vi "myRIO_BRig_RT__Case_Exp_State_Reward__v2.vi"(0 "input_dataCurrent":u16[](array[numeric]), 5 "input_state":T1, 9 "input_spout":enum16{"Left", "Right"}(ring), 12 "input_dataExp":u16[](array[numeric]), 13 "input_dataTrial":u16[][](array[numeric])) -> (4 "output_dataCurrent":u16[](array[numeric]), 6 "output_state":T1, 8 "output__L":bool, 10 "output__R":bool)   [LabVIEW 2014]
uses:
  myRIO_BRig_RT__Case_Exp_stateList.ctl
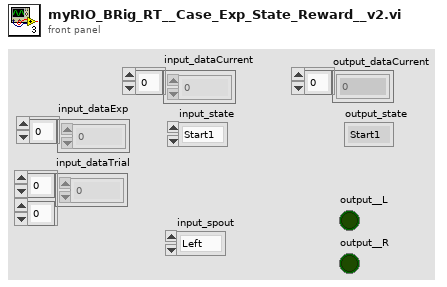
[diagram p1: front panel]
types:
  T1 = typedef "myRIO_BRig_RT__Case_Exp_stateList.ctl" = enum16{"Start1", "Start2", "Start3", "saveSettings1", "saveSettings2", "saveSettings3", "saveSettings4", "saveSettings_LC_ENL_l1", "saveSettings_LC_ENL_l2", "saveSettings_LC_Cue_l1", "saveSettings_LC_Cue_l2", "saveSettings6_LC_l1_Other", "SaveSettings6_LC_l2_Other", "setSettings_Audio", "setSettings_Laser", "initBlock_pre", "initBlock", "initBlock2", "initBlock_post", "initTrial_pre", "initTrial", "initTrial2", "initTrial3", "initTrial4", "initTrial_LC_ENL1", "initTrial_LC_Cue1", "initTrial_LC_Cue1_2", "initTrial_LC_Sel", "initTrial_post", "ENL1_pre", "ENL1", "ENL1_post", "ENL1Penalty_pre", "ENL1Penalty", "ENL2_pre", "ENL2", "ENL2Penalty_pre", "ENL2Penalty", "Cue1_pre", "Cue1", "Cue1_post", "Cue1Penalty_pre", "Cue1Penalty", "Cue2_pre", "Cue2", "Cue2Penalty_pre", "Cue2Penalty", "Selection_pre", "Selection", "Select_post", "SelectReward_pre", "SelectReward", "SelectRewardPost_pre", "SelectRewardPost", "SelectWrong_pre", "SelectWrong", "SelectWrong_post", "SelectTimeout_pre", "SelectTimeout", "SelectTimeout_post", "endTrial_pre", "endTrial1", "endTrial2", "endTrial3", "endTrial_post", "endBlock_pre", "endBlock", "endBlock_post", "endExp", "commConnect", "commUpload_pre", "commUpload_dataBlock", "commUpload_dataCurrent", "commUpload_dataExp", "commUpload_dataLC", "commUpload_dataTrial", "commUpload_post", "saveData_pre", "saveData_dataBlock", "saveData_dataCurrent", "saveData_dataExp", "saveData_dataLC", "saveData_dataTrial", "saveData_post", "empty_endBlock1", "empty_endBlock2", "empty_endTrial1", "empty_endTrial2", "empty_endTrial3", "empty_endTrial4", "empty_endTrial5", "dummyState", "dummyState_endBlock"}
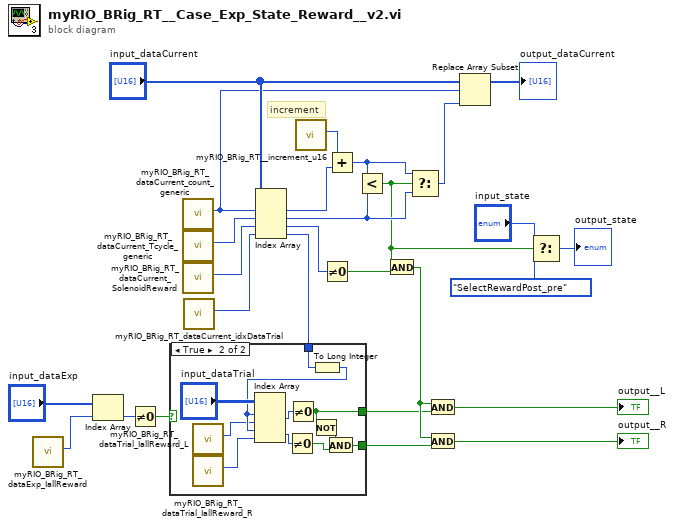
[diagram p0: block diagram]
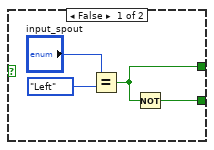
[diagram p2: hidden frame]
diagram:
  # "increment"
  n1 = call "myRIO_BRig_RT_dataExp_IallReward.vi"() -> ("output_I_allReward"=w7:i32)  [unwired: 11 in]
  n2 = Index Array(array="input_dataExp", index=w7) -> (element=w6:u16)
  n3 = Not Equal To 0?(x=w6) -> (x != 0?=w5:bool)
  n4 = call "myRIO_BRig_RT_dataCurrent_count_generic.vi"() -> ("output_count_generic"=w23:i32)  [unwired: 11 in]
  n5 = call "myRIO_BRig_RT_dataCurrent_Tcycle_generic.vi"() -> ("output_Tcycle_generic"=w25:i32)  [unwired: 11 in]
  n6 = call "myRIO_BRig_RT_dataCurrent_SolenoidReward.vi"() -> ("output_SolenoidReward"=w14:i32)  [unwired: 11 in]
  n7 = call "myRIO_BRig_RT_dataCurrent_idxDataTrial.vi"() -> ("output_idxDataTrial"=w2:i32)  [unwired: 11 in]
  n8 = Index Array(array="input_dataCurrent", index #1=w23, index #2=w25, index #3=w14, index #4=w2) -> (element #1=w24:u16, element #2=w22:u16, element #3=w13:u16, element #4=w1:u16)
  n9 = case shown="True" w5 {
    tunnel: [w28 w35] -> w4
    tunnel: [w29 w34] -> w3
    tunnel: w1 -> [_ w41]
    frame False {
      n10 = Equal?(x="input_spout", y=enum16{"Left", "Right"}."Left") -> (x = y?=w28:bool)
      n11 = Not(x=w28) -> (.not. x?=w29:bool)
    }
    frame True {
      n12 = call "myRIO_BRig_RT_dataTrial_IallReward_L.vi"() -> ("output_I_allReward_L"=w39:i32)  [unwired: 11 in]
      n13 = call "myRIO_BRig_RT_dataTrial_IallReward_R.vi"() -> ("output_I_allReward_R"=w38:i32)  [unwired: 11 in]
      n14 = To Long Integer(number=w41) -> (32bit integer=w40:i32)
      n15 = Index Array(array="input_dataTrial", index (row) #1=w40, index (col) #1=w39, index (row) #2=w40, index (col) #2=w38) -> (element #1=w37:u16, element #2=w36:u16)
      n16 = Not Equal To 0?(x=w36) -> (x != 0?=w32:bool)
      n17 = Not Equal To 0?(x=w37) -> (x != 0?=w35:bool)
      n18 = Not(x=w35) -> (.not. x?=w33:bool)
      n19 = And(x=w33, y=w32) -> (x .and. y?=w34:bool)
    }
  }
  n20 = call "myRIO_BRig_RT__increment_u16.vi"() -> ("output_increment__u16"=w19:u16)  [unwired: 11 in]
  n21 = Not Equal To 0?(x=w13) -> (x != 0?=w11:bool)
  n22 = Add(x=w19, y=w24) -> (x+y=w18:u16)
  n23 = Less?(x=w18, y=w22) -> (x < y?=w10:bool)
  n24 = And(x=w10, y=w11) -> (x .and. y?=w9:bool)
  n25 = Select(t=w18, s=w10, f=w22) -> (s? t:f=w21:u16)
  n26 = And(x=w9, y=w4) -> (x .and. y?=→"output__L":bool)
  n27 = And(x=w9, y=w3) -> (x .and. y?=→"output__R":bool)
  n28 = Replace Array Subset(array="input_dataCurrent", new element=w21, index=w23) -> (→"output_dataCurrent":u16[])
  n29 = Select(t="input_state", s=w10, f=myRIO_BRig_RT__Case_Exp_stateList."SelectRewardPost_pre" ("Enum")) -> (s? t:f=→"output_state":T1)
